vi "Create.vi"(8 "error in (no error)":errorcluster, 11 "Topic":string) -> (0 "error out":errorcluster, 3 "ViewerRef":T1)   [LabVIEW 2018, in "TopicViewer.lvlib"]
uses:
  TopicViewer.lvlib
  controls/viewewr_bus.ctl
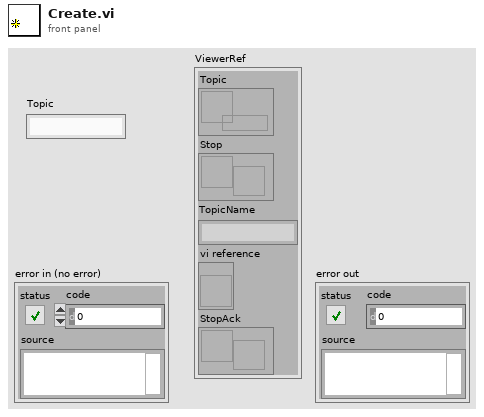
[diagram p1: front panel]
types:
  T1 = typedef "TopicViewer.lvlib/viewewr_bus.ctl" = cluster{"Topic":refnum<queue>, "Stop":refnum<notifier>, "TopicName":string, "vi reference":refnum<vi>, "StopAck":refnum<notifier>}
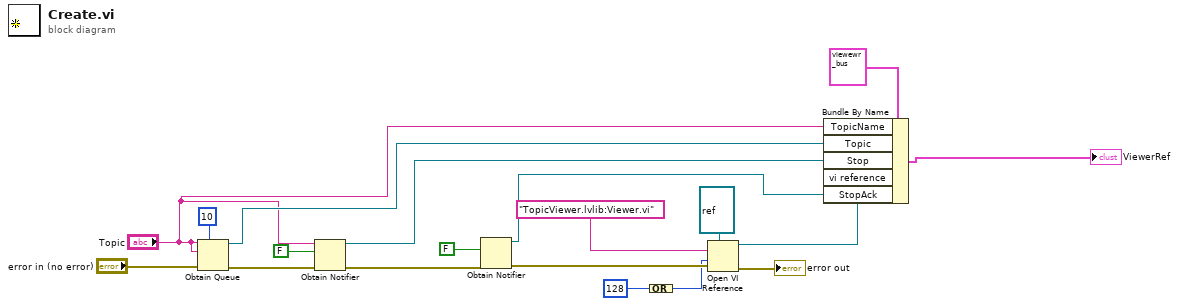
[diagram p0: block diagram]
diagram:
  n1 = Obtain Queue(max queue size (-1, unlimited)=10, name (unnamed)="Topic", element data type="Topic", error in (no error)="error in (no error)") -> (queue out=w15:refnum<queue>, error out=w18:errorcluster)  [unwired: 1 in, 1 out]
  n2 = Obtain Notifier(name (unnamed)="Topic", notification data type=FALSE, error in (no error)=w18) -> (notifier out=w14:refnum<notifier>, error out=w6:errorcluster)  [unwired: 1 in, 1 out]
  n3 = Obtain Notifier(notification data type=FALSE, error in (no error)=w6) -> (notifier out=w5:refnum<notifier>, error out=w4:errorcluster)  [unwired: 2 in, 1 out]
  n4 = Compound Arithmetic op=OR(128 ("options")) -> (w1:i32)
  n5 = Open VI Reference(type specifier VI Refnum (for type only)=refnum<vi> refnum, vi path="TopicViewer.lvlib:Viewer.vi", options=w1, error in (no error)=w4) -> (vi reference=w3:refnum<vi>, error out=→"error out":errorcluster)  [unwired: 2 in]
  n6 = Bundle By Name(cluster=T1 {"Topic"=refnum, "Stop"=refnum, "TopicName"="", "vi reference"=refnum, "StopAck"=refnum}, "TopicName"="Topic", "Topic"=w15, "Stop"=w14, "vi reference"=w3, "StopAck"=w5) -> (→"ViewerRef":T1)
